vi "Select a function.vi"(8 "error in (no error)":errorcluster, 10 "Function Name":string, 11 "Controller UI in":refnum<class "Controller UI.lvclass">) -> (0 "error out":errorcluster, 2 "success":bool, 3 "Controller UI out":refnum<class "Controller UI.lvclass">)   [LabVIEW 2016, in "Controller UI.lvlib" / "Controller UI.lvclass"]
uses:
  <userlib>/Common Components/Controller UI/Controller UI.lvclass
  <userlib>/Common Components/Controller UI/Controller UI.lvclass/Controller UI.ctl
  <userlib>/Common Components/Controller UI/Accessors/Read Function.vi
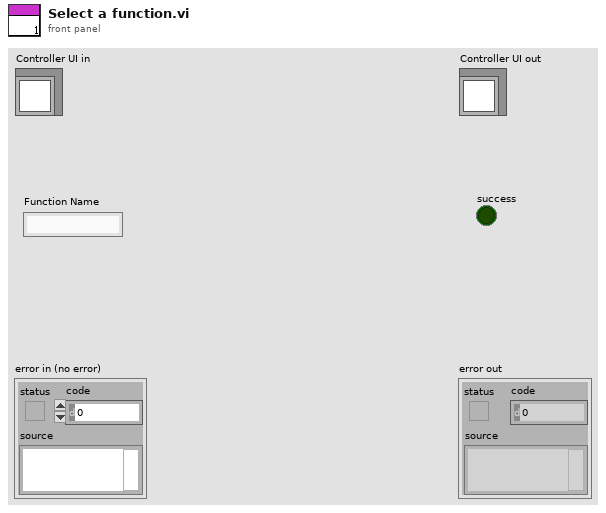
[diagram p1: front panel]
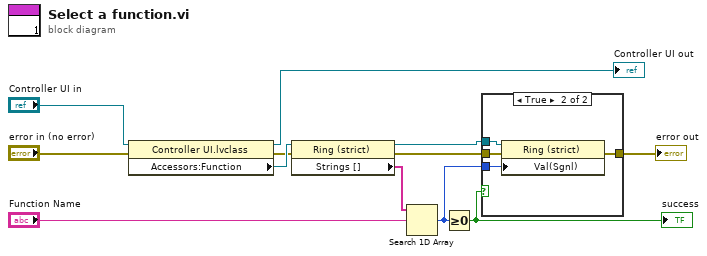
[diagram p0: block diagram]
diagram:
  n1 = property class="Controller UI.lvclass"(reference="Controller UI in", error in="error in (no error)") -> (reference out=→"Controller UI out":refnum<class "Controller UI.lvclass">, error out=w4:errorcluster, "Accessors:Function"=w10:refnum<vi>)
  n2 = property class="Ring (strict)"(reference=w10, error in=w4) -> (reference out=w7:refnum<vi>, error out=w3:errorcluster, "Strings []"=w9:string[])
  n3 = Search 1D Array(1D array=w9, element="Function Name") -> (index of element=w6:i32)  [unwired: 1 in]
  n4 = Greater Or Equal To 0?(x=w6) -> (x >= 0?=w1:bool)
  "success" <- w1
  n5 = case shown="True" w1 {
    tunnel: w7 -> [_ w17]
    tunnel: w6 -> [_ w16]
    tunnel: w3 -> [w13 w15]
    tunnel: [w13 w14] -> w2
    frame False {
    }
    frame True {
      n6 = property class="Ring (strict)"(reference=w17, error in=w15, "Val(Sgnl)"=w16) -> (error out=w14:errorcluster)  [unwired: 1 out]
    }
  }
  "error out" <- w2
